vi "Read General Setting from File.vi"(8 "error in (no error)":errorcluster) -> (0 "error out":errorcluster)   [LabVIEW 2015, in "ConfigHelper.lvlib"]
uses:
  ConfigHelper.lvlib
  Control_General Setup (Path).ctl
  Control_General Setup (String).ctl
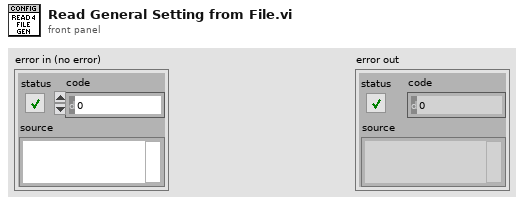
[diagram p1: front panel]
types:
  T1 = typedef "ConfigHelper.lvlib/Control_General Setup (Path).ctl" = cluster{"Export Path":path, "level":dbl, "Time Gap":dbl}
  T2 = typedef "ConfigHelper.lvlib/Control_General Setup (String).ctl" = cluster{"Export Path":string, "level":dbl, "Time Gap":dbl}
  T3 = typedef "PointValueMap.lvlib/PointMap.ctl" = refnum<data-value>
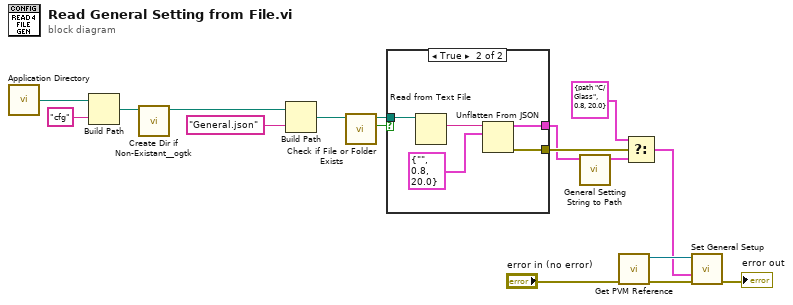
[diagram p0: block diagram]
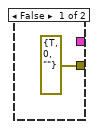
[diagram p2: hidden frame]
diagram:
  n1 = call <vilib>:"Application Directory.vi"() -> ("Application Directory"=w17:path)
  n2 = Build Path(base path=w17, name or relative path="cfg") -> (appended path=w15:path)
  n3 = call <userlib>:"Create Dir if Non-Existant__ogtk.vi"("Directory Path"=w15) -> ("dup Directory Path"=w14:path)  [unwired: 8 in, 2 out]
  n4 = Build Path(base path=w14, name or relative path="General.json") -> (appended path=w12:path)
  n5 = call <vilib>:"Check if File or Folder Exists.vi"("path"=w12) -> ("file or folder exists?"=w11:bool, "dup path"=w10:path)  [unwired: 8 in, 1 out]
  n6 = case shown="True" w11 {
    tunnel: w10 -> [_ w23]
    tunnel: [_ w20] -> w7
    tunnel: [errorcluster {"status"=TRUE, "code"=0, "source"=""} ("error constant") w19] -> w9
    frame False {
    }
    frame True {
      n7 = Read from Text File(file (use dialog)=w23) -> (text=w22:string)  [unwired: 3 in, 3 out]
      n8 = Unflatten From JSON(JSON string=w22, type and defaults=T2 {"Export Path"="", "level"=0.8, "Time Gap"=20.0} ("General Setup")) -> (value=w20:T2, error out=w19:errorcluster)  [unwired: 5 in]
    }
  }
  n9 = call "General Setting String to Path.vi"("General Setup (String)"=w7) -> ("General Setup (Path)"=w8:T1)  [unwired: 10 in]
  n10 = call "Get PVM Reference.vi"("error in (no error)"="error in (no error)") -> ("error out"=w4:errorcluster, "Map Out"=w5:T3)  [unwired: 9 in]
  n11 = Select(t=T1 {"Export Path"=path "C:/Glass", "level"=0.8, "Time Gap"=20.0} ("General Setup"), s=w9, f=w8) -> (s? t:f=w3:T1)
  n12 = call "Set General Setup.vi"("error in (no error)"=w4, "General Setup"=w3, "Map"=w5) -> ("error out"=→"error out":errorcluster)  [unwired: 7 in, 1 out]
